vi "Get Variant.vi"(8 "error in (no error)":errorcluster, 11 "int32 in":refnum<class "float.lvclass">) -> (0 "error out":errorcluster, 2 "Variant":variant, 3 "int32 out":refnum<class "float.lvclass">)   [LabVIEW 2020]
uses:
  float.lvclass
  float.lvclass/float.ctl
  E:/Labview/LV 2020/Libs/LV Protobuf Raw/Source/Proto Type Common/Proto Type Common.lvclass
  E:/Labview/LV 2020/Libs/LV Protobuf Raw/Source/Tag/Basic Type.lvclass
  E:/Labview/LV 2020/Libs/LV Protobuf Raw/Source/Proto Value/Proto Type.lvclass
  E:/Labview/LV 2020/Libs/LV Protobuf Raw/Source/Type Serializer/Type Serializer.lvclass
  E:/Labview/LV 2020/Libs/LV Protobuf Raw/Source/String Representable/String Representable.lvclass
  E:/Labview/LV 2020/Libs/LV Protobuf Raw/Source/Wire Type Group/Wire Type Group.lvclass
  E:/Labview/LV 2020/Libs/LV Protobuf Raw/Source/Scalar Encoder/Scalar Type.lvclass
  E:/Labview/LV 2020/Libs/LV Protobuf Raw/Source/I32 Encoder/I32.lvclass
  E:/Labview/LV 2020/Libs/LV Protobuf Raw/Source/float/float.lvclass
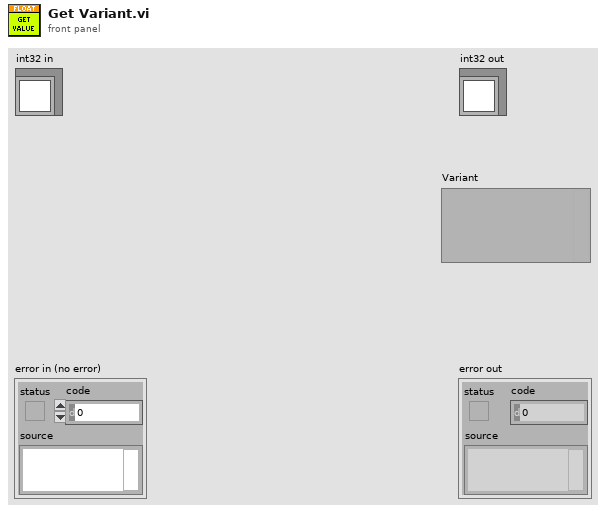
[diagram p1: front panel]
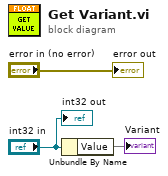
[diagram p0: block diagram]
diagram:
  n1 = Unbundle By Name("int32 in") -> ("Value"=→"Variant")
  "error out" <- "error in (no error)"
  "int32 out" <- "int32 in"
